vi "Color with Alpha.vi"(10 "Color":u32(colorbox), 11 "alpha":i32) -> (3 ".NET color Refnum out":refnum<k24>)   [LabVIEW 2015, in "Graph Extensions MSChart.lvlib"]
uses:
  Graph Extensions MSChart.lvlib
  System.Drawing
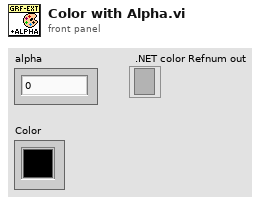
[diagram p1: front panel]
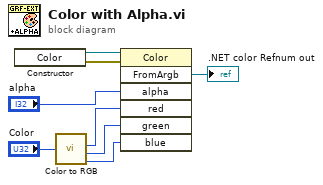
[diagram p0: block diagram]
diagram:
  n1 = constructor class="Color"() -> (reference out=w5:refnum<k24>, error out=w6:errorcluster)  [unwired: 3 in, 1 out]
  n2 = call <vilib>:"Color to RGB.vi"("Color"="Color") -> ("R"=w2:u8, "G"=w3:u8, "B"=w4:u8)  [unwired: 1 out]
  n3 = invoke class="Color" method="FromArgb"(reference=w5, error in=w6, "alpha"="alpha", "red"=w2, "green"=w3, "blue"=w4) -> ("FromArgb"=→".NET color Refnum out":refnum<k24>)  [unwired: 1 in, 6 out]
